vi "Algae Command.vi"(6 "Command Info In":T1, 7 "Negate or Confirm?":bool, 8 "Description":string, 9 "Setpoint":dbl, 10 "Algae State":T4=enum."Intake Algae", 11 "Operation":T5) -> (3 "Command Info Out":T1)   [LabVIEW 2023]
uses:
  Implementation/Algae Operations.ctl
  Support Code/Teleop Util/Algae States.ctl
  <vilib>/Rock Robotics/WPI/Framework/Command Status Info.ctl
  <vilib>/Rock Robotics/WPI/Framework/Completion Status.ctl
  <vilib>/Rock Robotics/WPI/Framework/Completion Notifier.ctl
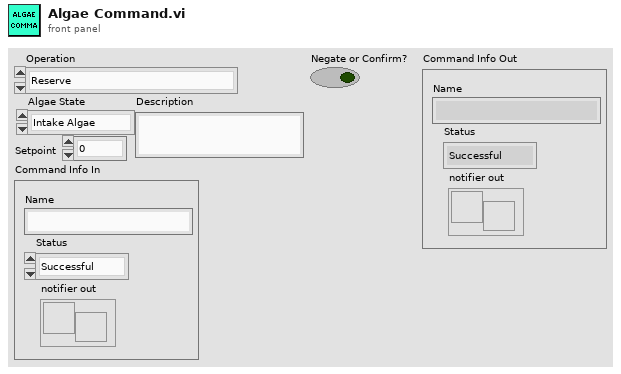
[diagram p1: front panel]
types:
  T1 = typedef "Command Status Info.ctl" = cluster{"Name":string, "Status":T2, "notifier out":T3}
  T2 = typedef "Completion Status.ctl" = enum16{"Successful", "Aborted", "Incomplete"}
  T3 = typedef "Completion Notifier.ctl" = refnum<notifier>
  T4 = typedef "Algae States.ctl" = enum16{"Idle", "Intake Algae", "Outtake Algae", "Stow", "Manual Overrides"}
  T5 = typedef "Algae Operations.ctl" = enum16{"Reserve", "Read Current", "Immediate", "Calibrate"}
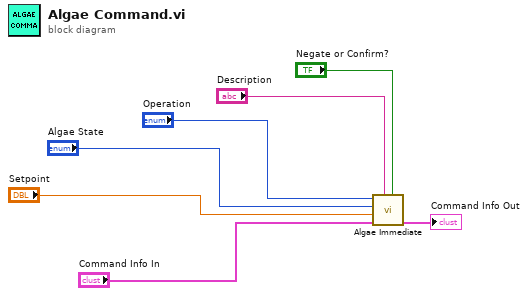
[diagram p0: block diagram]
diagram:
  n1 = call "Algae Immediate.vi"("Operation"="Operation", "Algae State"="Algae State", "Setpoint"="Setpoint", "Command Info In"="Command Info In", "Description"="Description", "Negate or Confirm?"="Negate or Confirm?") -> ("Command Info Out"=→"Command Info Out":T1)  [unwired: 4 in]
